vi "stop_sweep.vi"(8 "error in (no error)":errorcluster, 11 "DL090430TriggeredExperimentController in":refnum<class "ExperimentControllerDL090803Triggered.lvclass">) -> (0 "error out":errorcluster, 3 "DL090430TriggeredExperimentController out":refnum<class "ExperimentControllerDL090803Triggered.lvclass">)   [LabVIEW 2010, in "ExperimentControllerDL090803Triggered.lvclass"]
uses:
  ExperimentControllerDL090803Triggered.lvclass
  ImagingMode/GenericImagingMode/GenericImagingMode/GenericImagingMode.lvclass
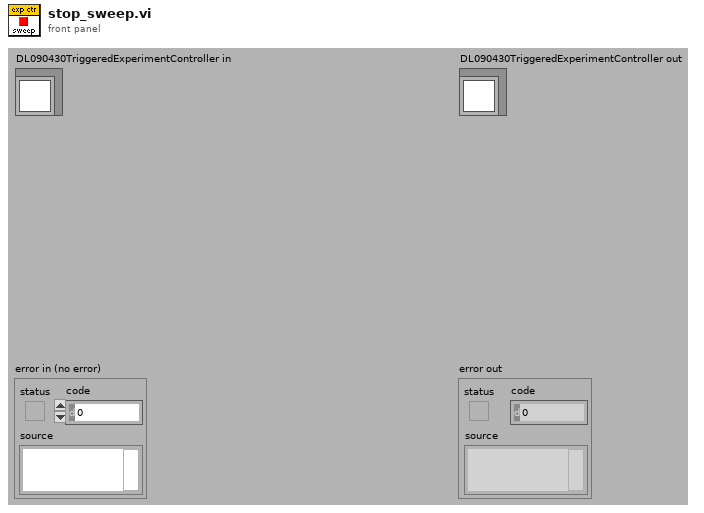
[diagram p1: front panel]
types:
  T1 = typedef "GenericToplevelComponent.lvclass/common_trigger_enum.ctl" = enum16{"NULL", "initialise", "terminate", "fetch command", "fetch data", "attach observer", "register as observer", "detach observer", "acknowledge", "start", "stop", "sweep started", "sweep finished", "experiment started", "experiment stopped"}
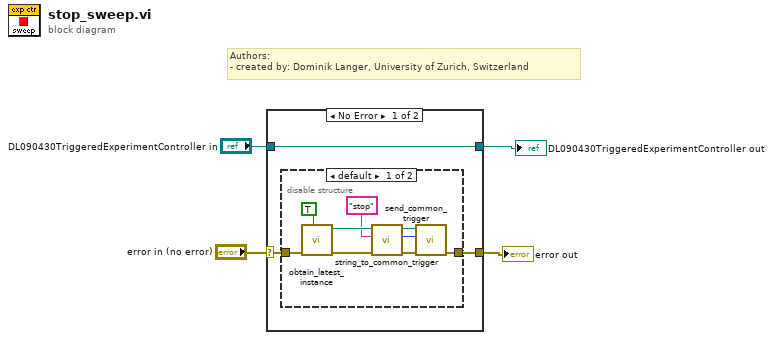
[diagram p0: block diagram]
diagram:
  # "Authors: \n- created by: Dominik Langer, University of Zurich, Switzerland"
  n1 = case shown="No Error" "error in (no error)" {
    selector: "error in (no error)" -> [w6 w19]
    tunnel: [w5 w19] -> w3
    tunnel: [w7 w18] -> w1
    tunnel: "DL090430TriggeredExperimentController in" -> [w7 w18]
    frame No Error {
      n2 = disable-structure shown="default" {
        disable-tunnel: w6 -> [w16 w17]
        disable-tunnel: [w15 w17] -> w5
        frame condition #0 (active) {
          n3 = call "obtain_latest_instance.vi"("quick, but maybe outdated?"=TRUE, "error in (no error)"=w16) -> ("error out"=w11:errorcluster, "GenericScanMode out"=w13:refnum<class "GenericImagingMode.lvclass">)  [unwired: 8 in]
          n4 = call-dynamic "string_to_common_trigger.vi"("error in (no error)"=w11, "trigger string"="stop", "GenericToplevelComponent in"=w13) -> ("error out"=w10:errorcluster, "trigger"=w9:T1, "GenericToplevelComponent out"=w12:refnum<class "GenericImagingMode.lvclass">)  [unwired: 6 in]
          n5 = call-dynamic "send_common_trigger.vi"("error in (no error)"=w10, "trigger"=w9, "GenericToplevelComponent in"=w12) -> ("error out"=w15:errorcluster)  [unwired: 6 in, 2 out]
        }
        frame condition #1 {
        }
      }
    }
    frame Error {
    }
  }
  "error out" <- w3
  "DL090430TriggeredExperimentController out" <- w1
